vi "TcpIp_SendMsg.vi"(10 "数据输入":string, 11 "连接ID":refnum<k5>) -> (3 "连接ID输出":refnum<k5>)   [LabVIEW 2013]
panel:
  out "错误输出":errorcluster
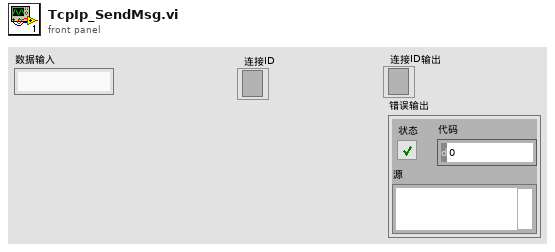
[diagram p1: front panel]
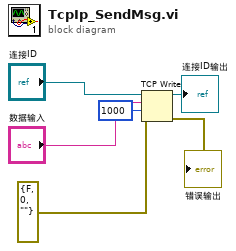
[diagram p0: block diagram]
diagram:
  n1 = TCP Write(connection ID="连接ID", data in="数据输入", error in (no error)=errorcluster {"status"=FALSE, "code"=0, "source"=""} ("错误输入（无错误）"), 9:1000 ("超时毫秒(25000)")) -> (connection ID out=→"连接ID输出":refnum<k5>, error out=→"错误输出":errorcluster)  [unwired: 1 out]
